vi "Checksum Update.vi"(11 "BGI Data In":string) -> (2 "old Checksum":string, 3 "BGI Data Out":string)   [LabVIEW 2019]
panel:
  out "checksum":string
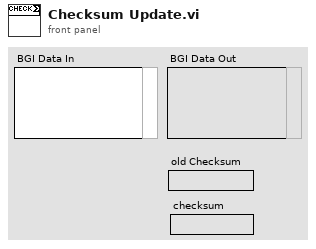
[diagram p1: front panel]
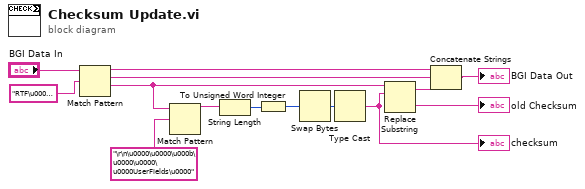
[diagram p0: block diagram]
diagram:
  n1 = Match Pattern(string="BGI Data In", regular expression="RTF\u0000\u0001\u0000\u0000\u0000" ("search string/char (-)")) -> (before substring=w8:string, match substring=w9:string, after substring=w4:string)  [unwired: 1 in, 1 out]
  n2 = Match Pattern(string=w4, regular expression="\r\n\u0000\u0000\u000b\u0000\u0000\u0000UserFields\u0000" ("search string/char (-)")) -> (before substring=w2:string)  [unwired: 1 in, 3 out]
  n3 = String Length(string=w2) -> (length=w1:i32)
  n4 = To Unsigned Word Integer(number=w1) -> (unsigned 16bit integer=w13:u16)
  n5 = Swap Bytes(anything=w13) -> (byte swapped=w14:u16)
  n6 = Type Cast(x=w14) -> (*(type *) &x=w10:string)  [unwired: 1 in]
  "checksum" <- w10
  n7 = Replace Substring(4:w10, 5:w4) -> (0:→"old Checksum":string, 1:w5:string)  [unwired: 2 in]
  n8 = Concatenate Strings(w8, w9, w5) -> (→"BGI Data Out":string)
